vi "DaqNavi test2.vi"() -> ()   [LabVIEW 2017]
uses:
  <userlib>/DAQNavi Polymorphic VI/create/DAQNavi Create Channel(AI-Voltage).vi
  <userlib>/DAQNavi Polymorphic VI/configure/timing/DAQNavi Timing(Convert Clock).vi
  <userlib>/DAQNavi Polymorphic VI/configure/DAQNavi Get Property/AI/DAQNaviGet_AI_ConvertClock_Rate.vi
  <userlib>/DAQNavi Polymorphic VI/read/DAQNavi Read (Analog 1D Wfm NChan NSamp).vi
panel:
  out "Waveform Graph":waveform(dbl)[](graph)
  in  "stop":bool
  out "value range  2":string="+/- 5 V" caption="property value"
  out "physical channels 2":string="DemoDevice,BID#0/ai0:1" caption="property value"
  out "convert rate 2":dbl
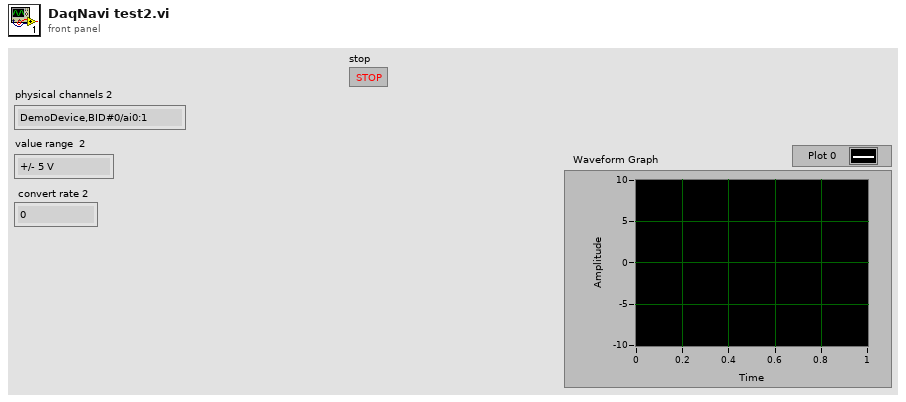
[diagram p1: front panel]
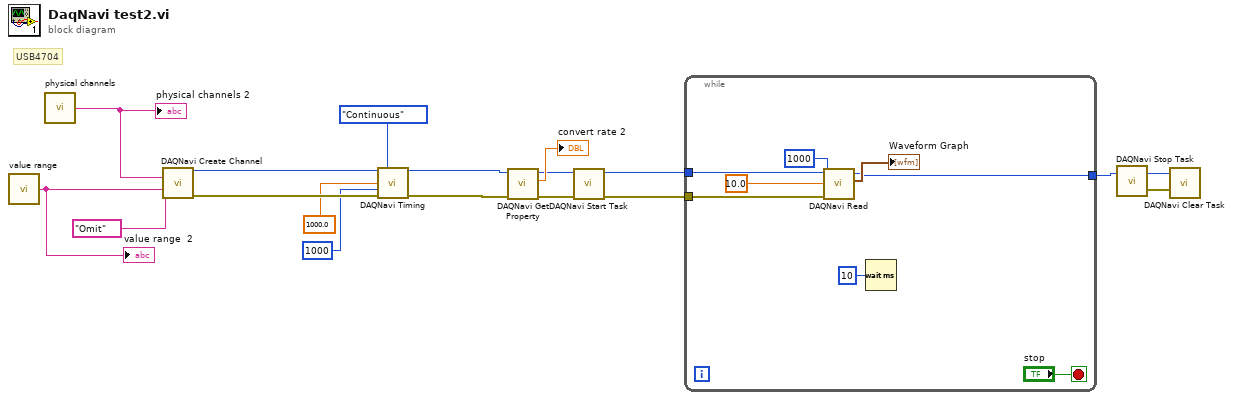
[diagram p0: block diagram]
diagram:
  # "USB4704"
  n1 = call "value range"() -> ("property value"=w18:string)  [unwired: 1 out]
  "value range  2" <- w18
  n2 = call "physical channels"() -> ("property value"=w4:string)  [unwired: 1 out]
  "physical channels 2" <- w4
  n3 = call-poly <userlib>:"DAQNavi Create Channel.vi"("physical channels"=w4, "signal type"="Omit", "value range"=w18) -> ("task out"=w12:i32, "error out"=w13:errorcluster)  [unwired: 2 in, 9 out]
  n4 = call-poly <userlib>:"DAQNavi Timing.vi"("task in"=w12, "sample mode"=enum16{"Finite", "Continuous"}."Continuous", "rate"=1000.0, "samples per channel"=u32 1000, "error in (no error)"=w13) -> ("task out"=w15:i32, "error out"=w16:errorcluster)  [unwired: 1 in, 8 out]
  n5 = call-poly <userlib>:"DAQNavi Get Property.vi"("error in (no error)"=w16, "task in"=w15) -> ("error out"=w8:errorcluster, "rate"=→"convert rate 2":dbl, "task out"=w9:i32)  [unwired: 7 out]
  n6 = call <userlib>:"DAQNavi Start Task.vi"("error in (no error)"=w8, "task in"=w9) -> ("error out"=w6:errorcluster, "task out"=w7:i32)  [unwired: 8 in]
  n7 = while {
    tunnel: w7 -> [w26]
    tunnel: w6 -> [w25]
    tunnel: [w19] -> w3
    stop <- "stop" stop-if-true
    n8 = call-poly <userlib>:"DAQNavi Read.vi"("error in (no error)"=w25, "number of samples per channel to read"=u32 1000, "timeout"=10.0, "task in"=w26) -> ("data"=→"Waveform Graph":waveform(dbl)[], "task out"=w19:i32)  [unwired: 6 out]
    n9 = Wait (ms)(milliseconds to wait=u32 10) -> ()  [unwired: 1 out]
  }
  n10 = call <userlib>:"DAQNavi Stop Task.vi"("task in"=w3) -> ("error out"=w2:errorcluster, "task out"=w1:i32)  [unwired: 1 in]
  n11 = call <userlib>:"DAQNavi Clear Task.vi"("error in (no error)"=w2, "task in"=w1) -> ()  [unwired: 1 in, 1 out]
